vi "Acquire Sensor Data.vi"(8 "error in (no error)":errorcluster, 10 "Test Channel Map":variant, 11 "Sensor Parameter in":refnum<class "Sensor Parameter.lvclass">) -> (0 "error out":errorcluster, 3 "Sensor Parameter out":refnum<class "Sensor Parameter.lvclass">)   [LabVIEW 2013, in "Parameter.lvlib" / "Sensor Parameter.lvclass"]
uses:
  Sensor Parameter.lvclass
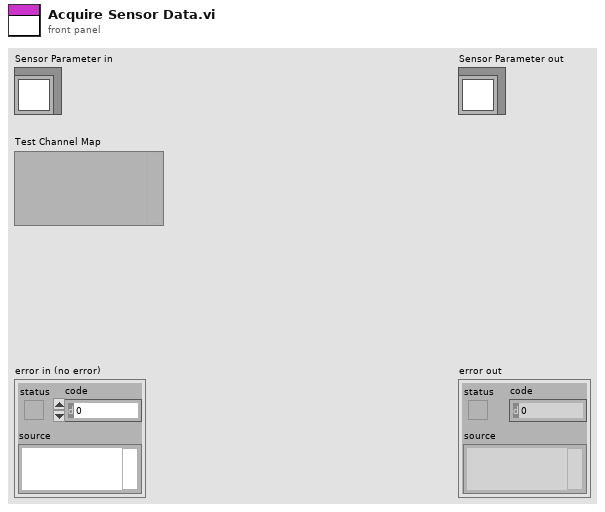
[diagram p1: front panel]
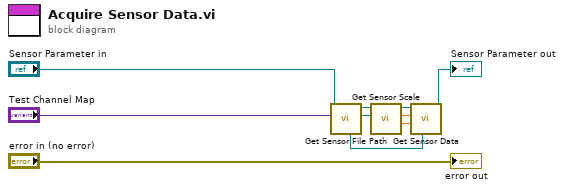
[diagram p0: block diagram]
diagram:
  n1 = call "Get Sensor File Path.vi"("Test Channel Map"="Test Channel Map", "Sensor Parameter in"="Sensor Parameter in") -> ("Sensor File Path"=w7:path, "Sensor Parameter out"=w8:refnum<class "Sensor Parameter.lvclass">, "Test Channel Path"=w1:path)  [unwired: 6 in, 1 out]
  n2 = call "Get Sensor Scale.vi"("Sensor File Path"=w7, "Sensor Parameter in"=w8) -> ("Intercept"=w4:dbl, "Slope"=w5:dbl, "Sensor Parameter out"=w6:refnum<class "Sensor Parameter.lvclass">)  [unwired: 6 in, 1 out]
  n3 = call "Get Sensor Data.vi"("Test Channel Path"=w1, "Intercept"=w4, "Slope"=w5, "Sensor Parameter in"=w6) -> ("Sensor Parameter out"=→"Sensor Parameter out":refnum<class "Sensor Parameter.lvclass">)  [unwired: 6 in, 1 out]
  "error out" <- "error in (no error)"
